vi "Read Current (List Voltage Sweep).vi"(5 "Delay Time (0.5 S)":dbl=0.5, 7 "Sweep Points (5)":i32=5, 8 "error in (no error)":errorcluster, 9 "Sweep List (V)":dbl[](array[numeric]), 10 "Source Measure Unit Channel (0: Channel A)":i32(ring) items=["Channel A", "Channel B"], 11 "VISA resource name":refnum<visa-resource-name>) -> (0 "error out":errorcluster, 2 "Current (A)":dbl[](array[numeric]), 3 "VISA resource name out":refnum<visa-resource-name>)   [LabVIEW 2020, in "Keithley 2600 Series.lvlib"]
doc: "Performs a voltage list sweep with current measured at every point."
uses:
  Keithley 2600 Series.lvlib
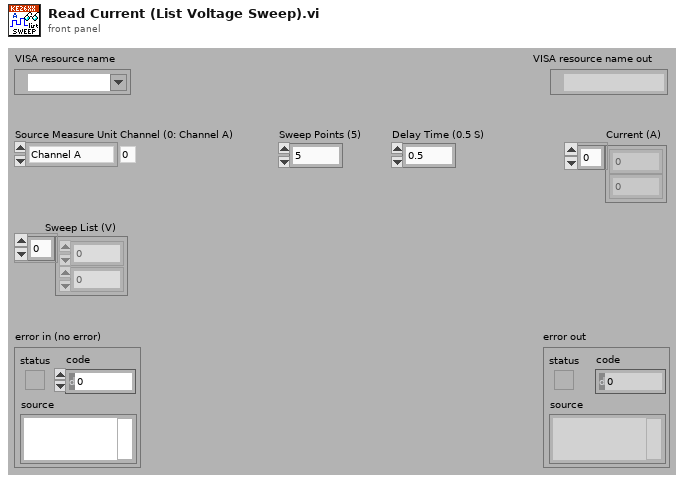
[diagram p1: front panel]
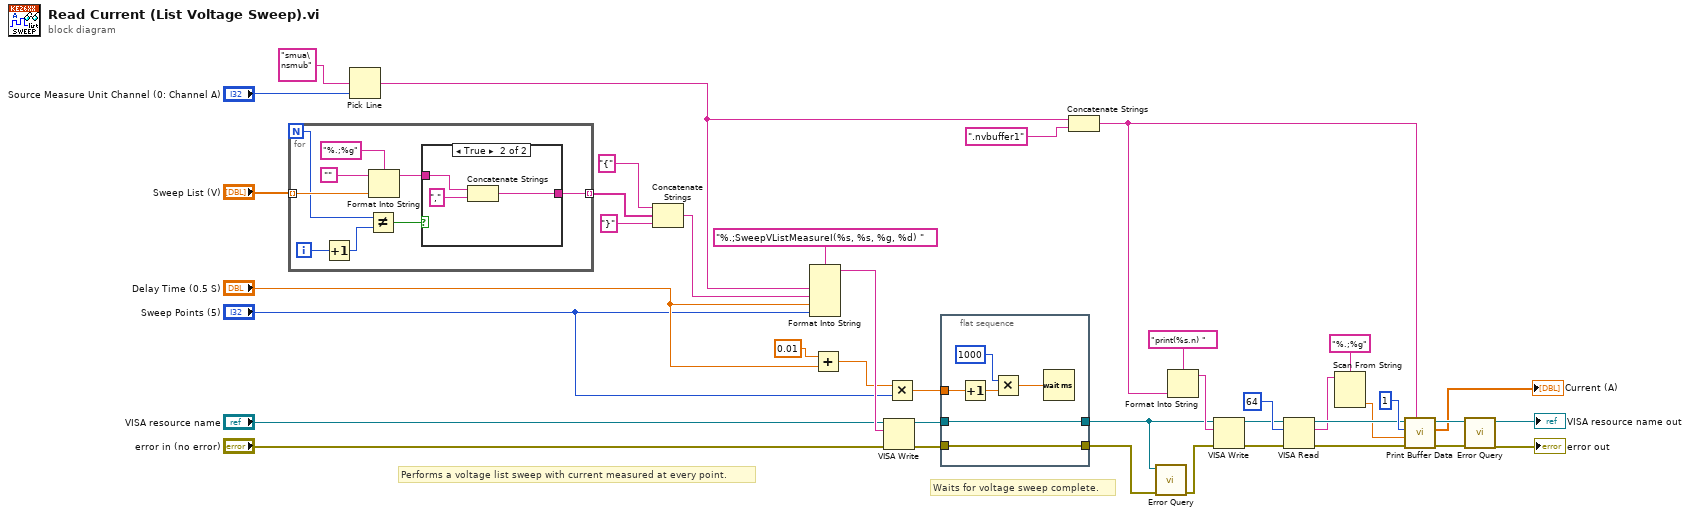
[diagram p0: block diagram]
diagram:
  # "Waits for voltage sweep complete."
  # "Performs a voltage list sweep with current measured at every point."
  n1 = for {
    N -> [w41]
    tunnel: "Sweep List (V)" -> [w49] mode=indexing
    tunnel: [w42] -> w32 mode=indexing
    i -> [w46]
    n2 = Increment(x=w46) -> (x+1=w45:i32)
    n3 = Not Equal?(x=w41, y=w45) -> (x != y?=w44:bool)
    n4 = Format Into String(format string="%.;%g", initial string="", w49) -> (resulting string=w43:string)  [unwired: 1 in, 1 out]
    n5 = case shown="True" w44 {
      tunnel: w43 -> [w50 w53]
      tunnel: [w50 w51] -> w42
      frame False {
      }
      frame True {
        n6 = Concatenate Strings(w53, ",") -> (w51:string)
      }
    }
  }
  n7 = Pick Line(multi-line string="smua\nsmub", line index="Source Measure Unit Channel (0: Channel A)") -> (output string=w7:string)  [unwired: 1 in]
  n8 = Concatenate Strings("{" ("string"), w32, "}") -> (w29:string)
  n9 = Format Into String(format string="%.;SweepVListMeasureI(%s, %s, %g, %d) ", w7, w29, "Delay Time (0.5 S)", "Sweep Points (5)") -> (resulting string=w39:string)  [unwired: 2 in, 1 out]
  n10 = Add(x=0.01, y="Delay Time (0.5 S)") -> (x+y=w23:dbl)
  n11 = VISA Write(VISA resource name="VISA resource name", write buffer=w39, error in (no error)="error in (no error)") -> (VISA resource name out=w27:refnum<visa-resource-name>, error out=w26:errorcluster)  [unwired: 1 out]
  n12 = Multiply(x=w23, y="Sweep Points (5)") -> (x*y=w21:dbl)
  n13 = flat-sequence {
    tunnel: w27 -> [w59]
    tunnel: w26 -> [w58]
    tunnel: [w59] -> w1
    tunnel: [w58] -> w3
    tunnel: w21 -> [w57]
    frame #0 {
      n14 = Increment(x=w57) -> (x+1=w56:dbl)
      n15 = Multiply(x=1000, y=w56) -> (x*y=w54:dbl)
      n16 = Wait (ms)(milliseconds to wait=w54) -> ()  [unwired: 1 out]
    }
  }
  n17 = Concatenate Strings(w7, ".nvbuffer1" ("string")) -> (w8:string)
  n18 = call "Error Query.vi"("error in (no error)"=w3, "VISA resource name"=w1) -> ("error out"=w2:errorcluster)  [unwired: 6 in, 3 out]
  n19 = Format Into String(format string="print(%s.n) ", w8) -> (resulting string=w10:string)  [unwired: 2 in, 1 out]
  n20 = VISA Write(VISA resource name=w1, write buffer=w10, error in (no error)=w2) -> (VISA resource name out=w13:refnum<visa-resource-name>, error out=w12:errorcluster)  [unwired: 1 out]
  n21 = VISA Read(VISA resource name=w13, byte count=u32 64, error in (no error)=w12) -> (VISA resource name out=w18:refnum<visa-resource-name>, read buffer=w16:string, error out=w17:errorcluster)  [unwired: 1 out]
  n22 = Scan From String(format string="%.;%g", input string=w16) -> (output 1=w15:dbl)  [unwired: 3 in, 3 out]
  n23 = call "Print Buffer Data.vi"("Reading Buffer (smua.nvbuffer1)"=w8, "error in (no error)"=w17, "End Index (1)"=w15, "Start Index (1)"=1 ("Start Index (0)"), "VISA resource name"=w18) -> ("error out"=w5:errorcluster, "Buffer Data"=→"Current (A)":dbl[], "VISA resource name out"=w6:refnum<visa-resource-name>)  [unwired: 4 in]
  n24 = call "Error Query.vi"("error in (no error)"=w5, "VISA resource name"=w6) -> ("error out"=→"error out":errorcluster, "VISA resource name out"=→"VISA resource name out":refnum<visa-resource-name>)  [unwired: 6 in, 2 out]
